vi "GUID_Test_Write&Read.vi"() -> ()   [LabVIEW 2018]
panel:
  out ".NET GUID":string
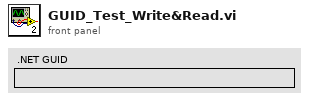
[diagram p1: front panel]
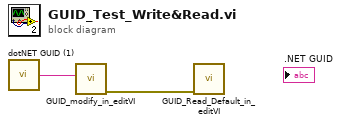
[diagram p0: block diagram]
diagram:
  n1 = call "dotNET GUID (1).vi"() -> (".NET GUID"=w2:string)
  n2 = call "GUID_modify_in_editVI.vi"(".NET GUID"=w2) -> ("error out"=w1:errorcluster)  [unwired: 10 in]
  n3 = call "GUID_Read_Default_in_editVI.vi"("error in (no error)"=w1) -> ()  [unwired: 7 in, 4 out]
